vi "Main_12A.vi"() -> ()   [LabVIEW 2024]
uses:
  Utility/Universal Utility/TypeDefs_Utility/Cluster_Row-Column.ctl
  <vilib>/Utility/miscctls.llb/LVMapReplaceAction.ctl
panel:
  out "Map 2":map{string, map{T1, u32}[]}(c390)
  out "Area":i32[](array[numeric])
  out "Plant Array":string[](array[string])
  out "Perimeter":u32[](array[numeric])
  in  "Example 3":string="RRRRIICCFF\nRRRRIICCCF\nVVRRRCCFFF\nVVRCCCJFFF\nVVVVCJJCFE\nVVIVCCJJEE\nVVIIICJJEE\nMIIIIIJJEE\nMIIISIJEEE\nMMMISSJEEE"
  in  "Example 2":string="OOOOO\nOXOXO\nOOOOO\nOXOXO\nOOOOO"
  in  "Use Puzzle":bool
  out "Answer 1371306":u32
  in  "Puzzle":string="WWWWWWWWWWWWWWWWWWHHHHHHHHHHHBYYYYYYYYYYYJJJJJJJJJJJJJJZLLLLLLLLLLLLLLLLLLLLLLBBYBBBBBBBBTTTTKKKKKKKKKKKKKOOOUUUUUUUUUUUSSSSSSSSSSSSSSSSSSSO\nWWWWWWWWWWWWWWWWWWHEHEHHHHHHBBBYYYYYYYYYYJJJJJJJWJJZJZZZZLLLLLLLLLLLLLLLLLLLLLBBBBBBBBBBBBTTTKKKKKKKKKKKKKOOOUUUUUUUUUUUUSSSSSSSSSSSSSSSSSHH\nWWWWWWWWWWWWWWWWWWWEEEHHHHHBBBBBYYYYYYYYYJYJJJJWWJJZZZZZZLLLFFFLLLFLLLHHHHHHHLBBBBBBBBBBBBTTTKKKKKKKKKKKKKOOOOUUUUUUUUUSSSSSSSSSSSSSSSSSSSHH\nWWWWWWWWWWWWWWWWWEEEEEEEEHHBBBSSYYYYYYYYYYYWWWWWWJJZZZZZZLFLFFFFFLFFFLHHHNHHHHABBBBBBBBBBBTTKKKKKKKKKKKKKKOOOUUUUUUUUUUSSSSSSSSSSSSSSSSSHHHH\nWWWWWWWWWWWWWWGEEEEEEEEHEHHHHHHSYYYY..."
  in  "Example 1":string="AAAA\nBBCD\nBBCC\nEEEC"
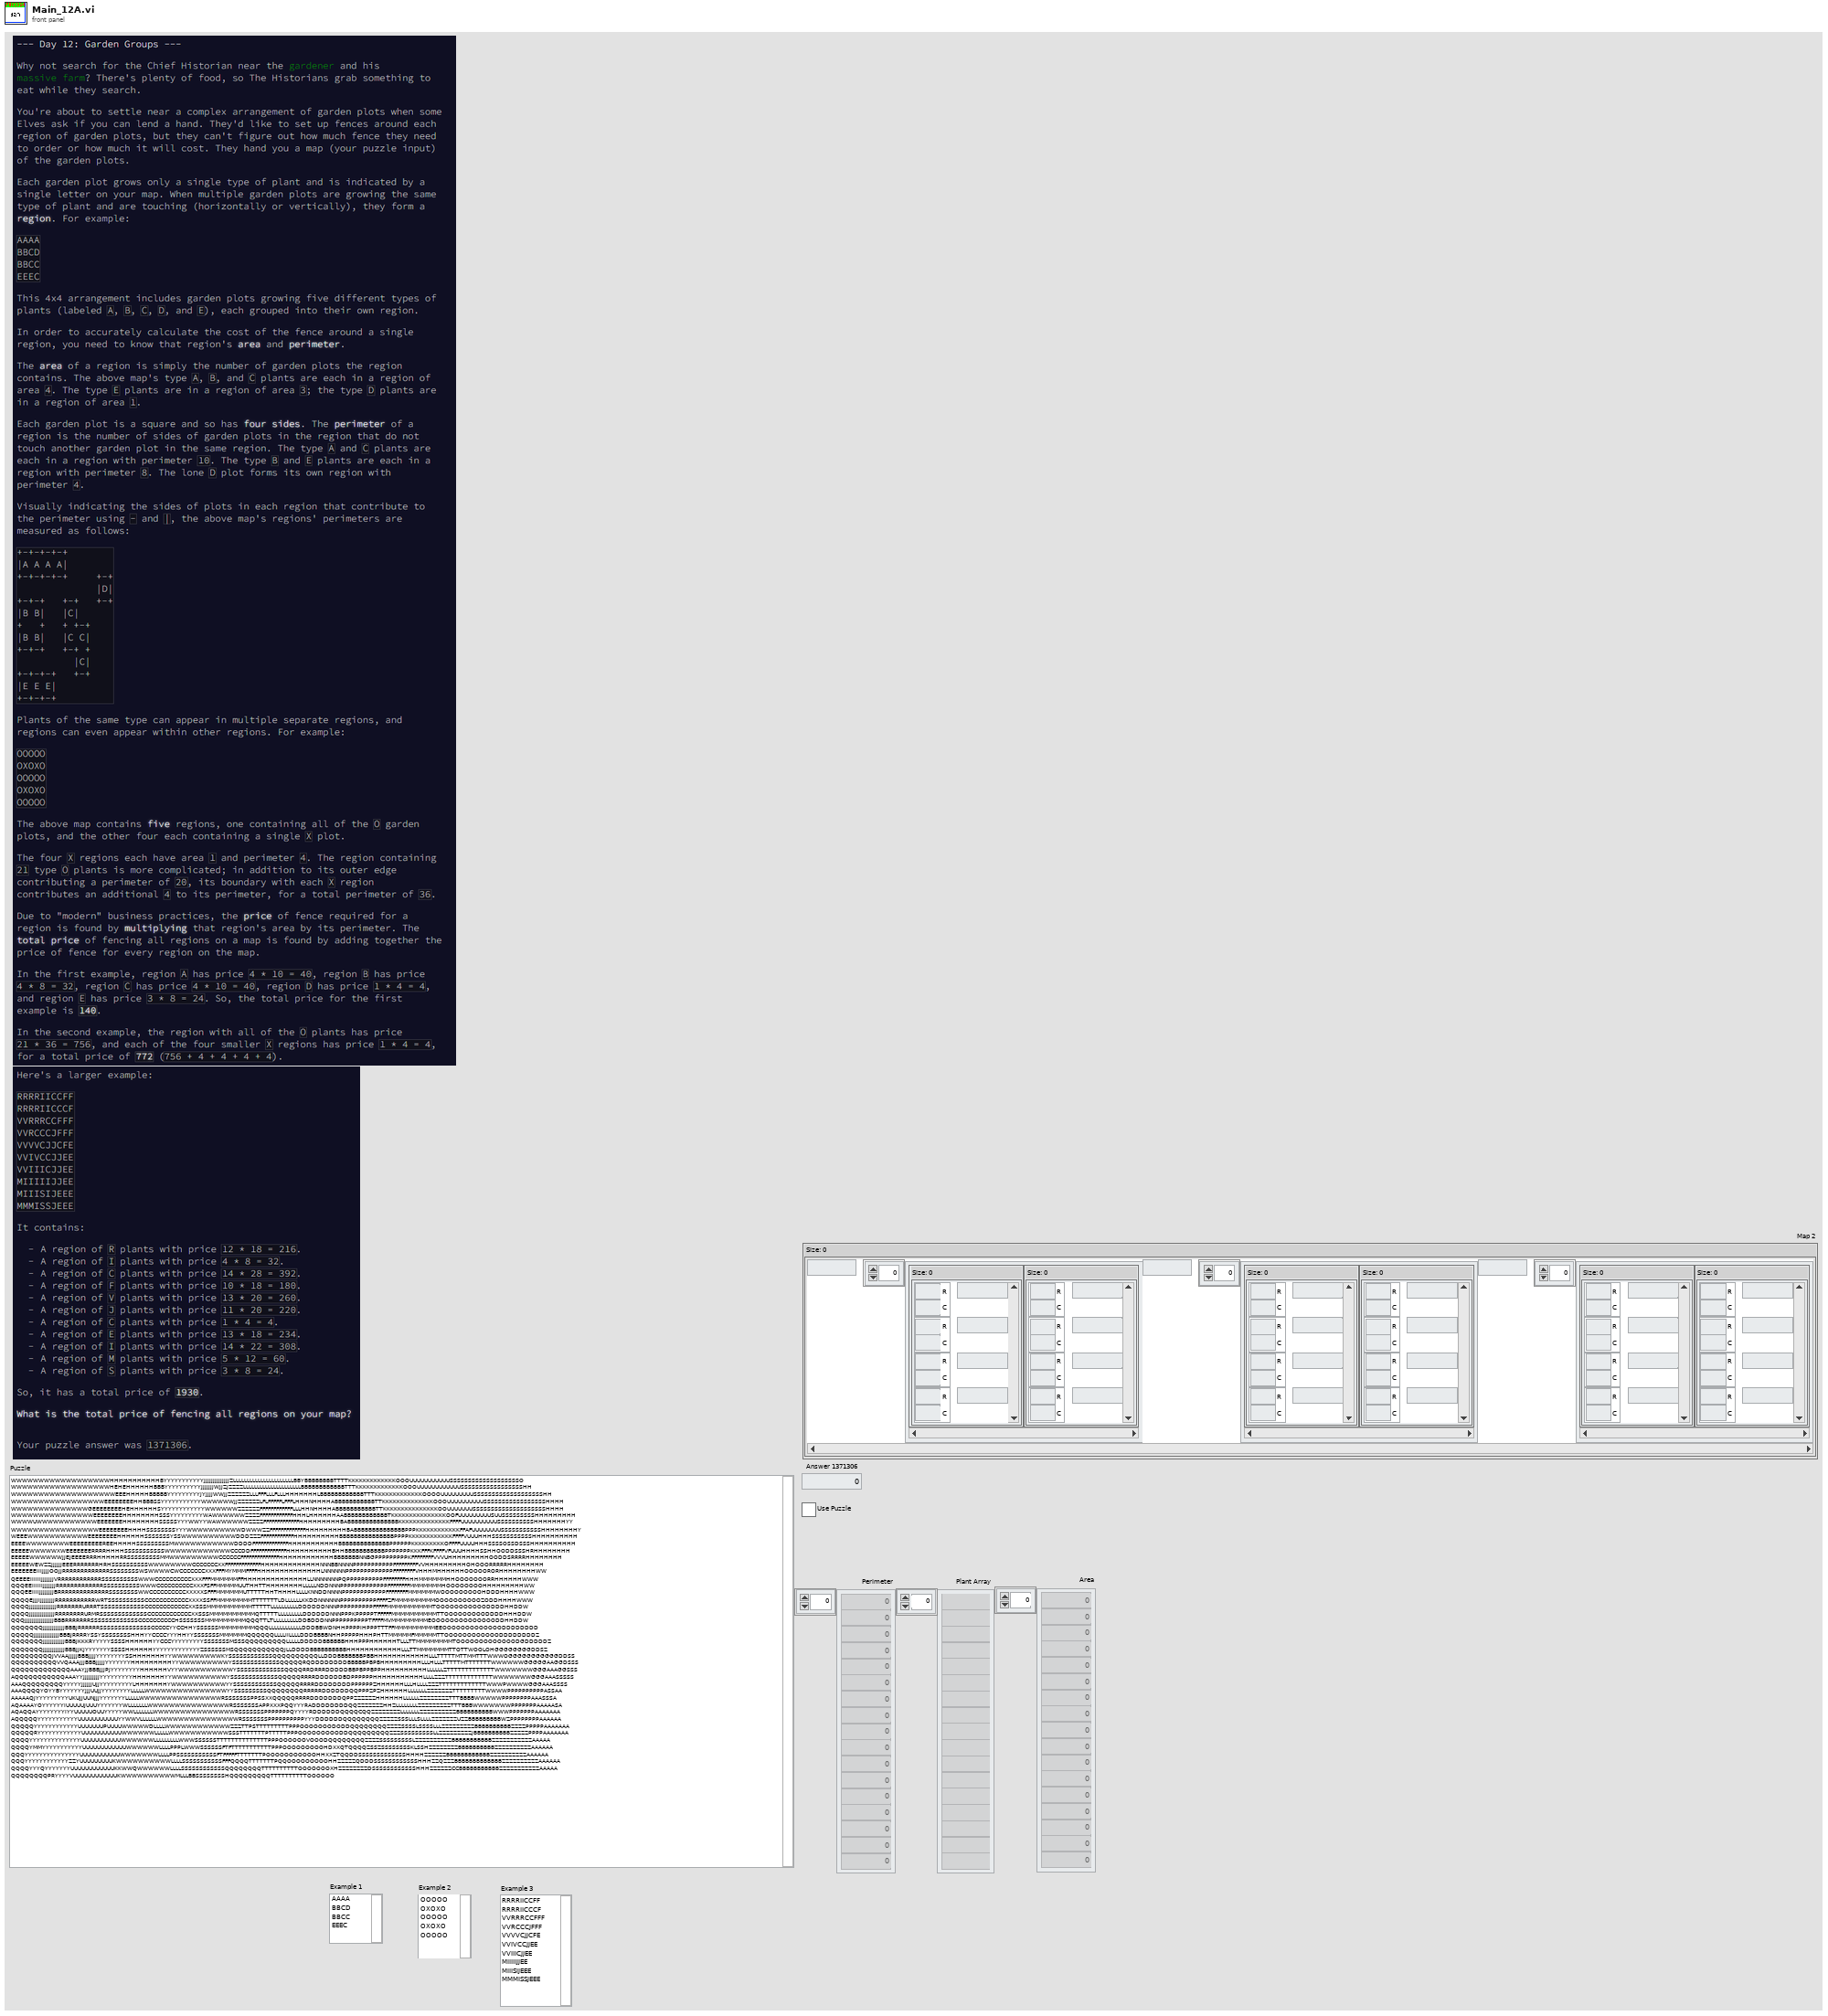
[diagram p1: front panel]
types:
  T1 = typedef "Cluster_Row-Column.ctl" = cluster{"R":i32, "C":i32}
  T2 = typedef "LVMapReplaceAction.ctl" = enum32{"Modify Entry only if found", "Add or Modify Entry", "Delete Entry"}
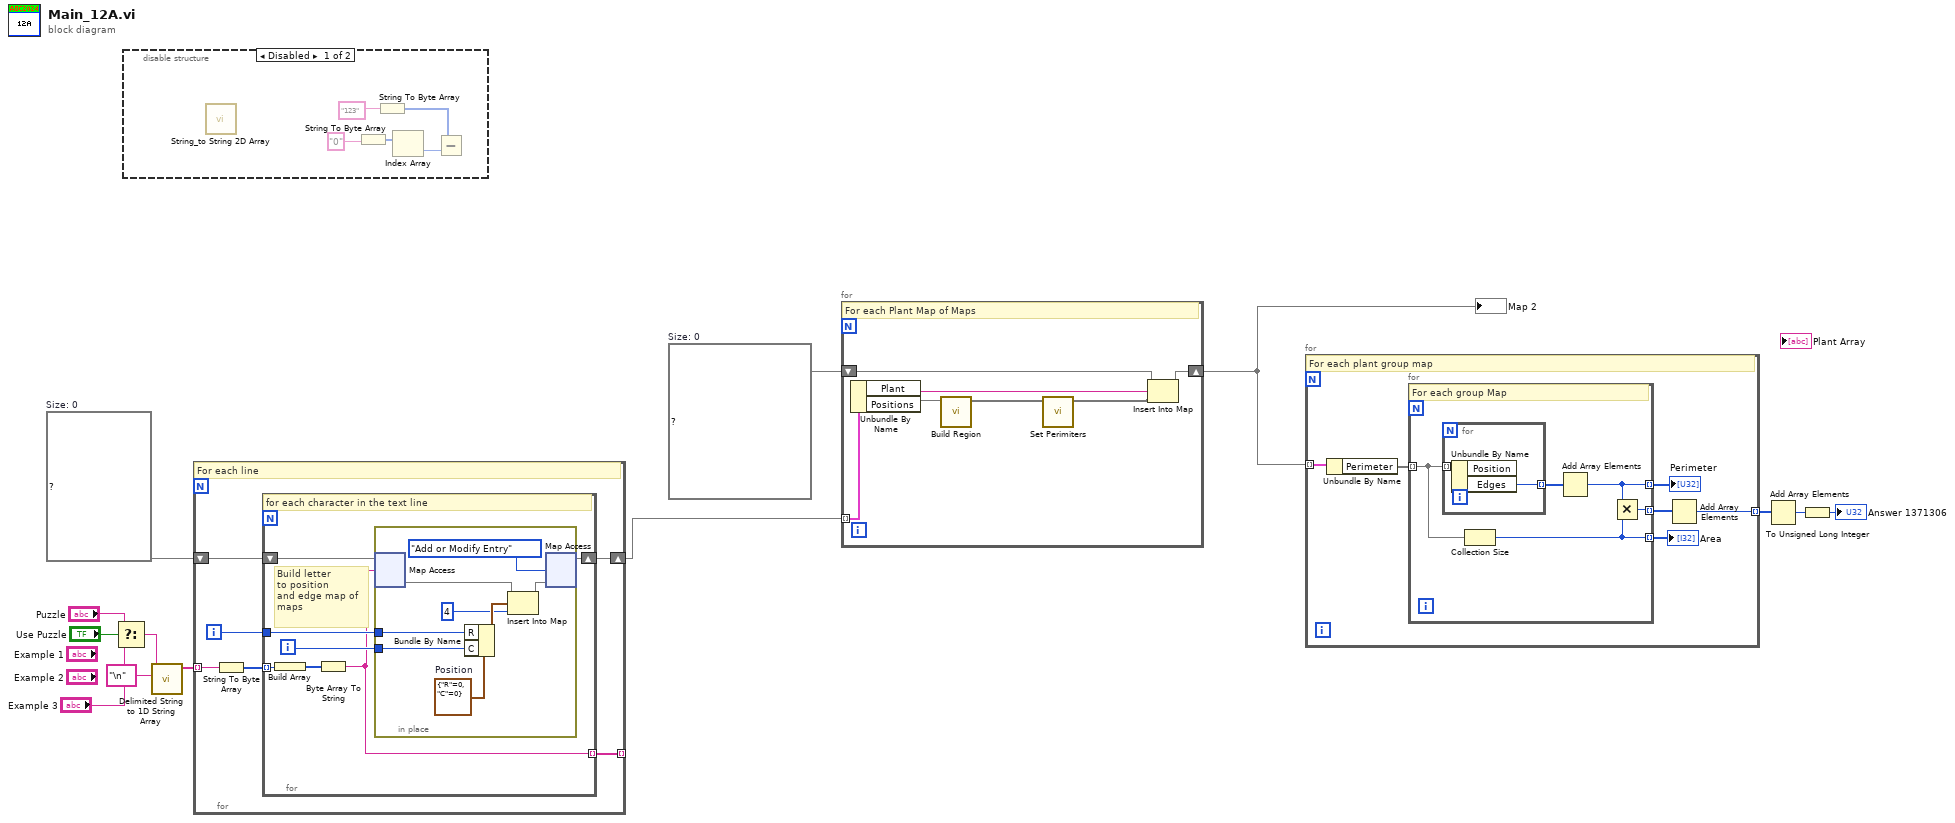
[diagram p0: block diagram]
diagram:
  w6 = map{string, map{T1, u32}[]} {}  # Size: 0
  w8 = map{string, map{T1, u32}} {}  # Size: 0
  n1 = Select(t="Puzzle", s="Use Puzzle", f="Example 3") -> (s? t:f=w11:string)
  n2 = disable-structure shown="Disabled" {
    frame Disabled {
      n3 = call "String_to String 2D Array.vi"() -> ()  [unwired: 11 in, 1 out]
      n4 = String To Byte Array(string="0") -> (unsigned byte array=w16:u8[])
      n5 = String To Byte Array(string="123") -> (unsigned byte array=w14:u8[])
      n6 = Index Array(array=w16) -> (element=w15:u8)  [unwired: 1 in]
      n7 = Subtract(x=w14, y=w15) -> ()  [unwired: 1 out]
    }
    frame Enabled {
    }
  }
  n8 = call <vilib>:"Delimited String to 1D String Array.vi"("delimiter"="\n" ("delimiter (Tab)"), "delimited string"=w11) -> ("string array"=w12:string[])  [unwired: 9 in]
  n9 = for {
    tunnel: w12 -> [w24] mode=indexing
    shift-right: [w21] -> w7
    shift-left: w8 -> [w22]
    tunnel: [w19] -> _ mode=indexing
    i -> [w20]
    # "For each line"
    n10 = String To Byte Array(string=w24) -> (unsigned byte array=w23:u8[])
    n11 = for {
      tunnel: w23 -> [w31] mode=indexing
      shift-right: [w28] -> w21
      shift-left: w22 -> [w29]
      tunnel: w20 -> [w27]
      tunnel: [w25] -> w19 mode=indexing
      i -> [w26]
      # "Build letter\nto position\nand edge map of\nmaps"
      # "for each character in the text line"
      n12 = Build Array(w31) -> (w30:u8[])
      n13 = Byte Array To String(unsigned byte array=w30) -> (string=w25:string)
      n14 = in-place {
        in-place-border: w27 -> [w37]
        in-place-border: w26 -> [w36]
        w38 = T1 {"R"=0, "C"=0}  # Position
        n15 = in-place-map #1(w29, w25) -> (w35:map{T1, u32})  [unwired: 1 in, 1 out]
        n16 = Bundle By Name(cluster=w38, "R"=w37, "C"=w36) -> (w33:T1)
        n17 = Insert Into Map(map in=w35, key=w33, value=u32 4) -> (map out=w34:map{T1, u32})  [unwired: 2 out]
        n18 = in-place-map #1(w34, LVMapReplaceAction."Add or Modify Entry" ("action")) -> (w28:map{string, map{T1, u32}})  [unwired: 2 out]
      }
    }
  }
  n19 = for {
    tunnel: w7 -> [w46] mode=indexing
    shift-right: [w44] -> w5
    shift-left: w6 -> [w45]
    # "For each Plant Map of Maps"
    n20 = Unbundle By Name(w46) -> ("Plant"=w43:string, "Positions"=w42:map{T1, u32})
    n21 = call "Build Region.vi"("Plant Positions"=w42) -> ("Plant Regions"=w41:map{T1, u32}[])  [unwired: 10 in]
    n22 = call "Set Perimiters.vi"("Plant Regions"=w41) -> ("Plant Regions 2"=w40:map{T1, u32}[])  [unwired: 10 in]
    n23 = Insert Into Map(map in=w45, key=w43, value=w40) -> (map out=w44:map{string, map{T1, u32}[]})  [unwired: 2 out]
  }
  "Map 2" <- w5
  n24 = for {
    tunnel: w5 -> [w52] mode=indexing
    tunnel: [w49] -> w4 mode=indexing
    # "For each plant group map"
    n25 = Unbundle By Name(w52) -> ("Perimeter"=w51:map{T1, u32}[])
    n26 = for {
      tunnel: w51 -> [w57] mode=indexing
      tunnel: [w55] -> w48 mode=indexing
      tunnel: [w54] -> w47 mode=indexing
      tunnel: [w53] -> w50 mode=indexing
      # "For each group Map"
      n27 = for {
        tunnel: w57 -> [w59] mode=indexing
        tunnel: [w58] -> w56 mode=indexing
        n28 = Unbundle By Name(w59) -> ("Edges"=w58:u32)  [unwired: 1 out]
      }
      n29 = Collection Size(1:w57) -> (0:w54:i32)
      n30 = Add Array Elements(numeric array=w56) -> (sum=w55:u32)
      n31 = Multiply(x=w55, y=w54) -> (x*y=w53:u32)
    }
    "Perimeter" <- w48
    "Area" <- w47
    n32 = Add Array Elements(numeric array=w50) -> (sum=w49:u32)
  }
  n33 = Add Array Elements(numeric array=w4) -> (sum=w3:u32)
  n34 = To Unsigned Long Integer(number=w3) -> (unsigned 32bit integer=→"Answer 1371306":u32)
